vi "Brick setting.vi"(5 "stage":i32, 7 "Ref_brick":refnum<vi>[](array[refnum])) -> (0 "brick(s)":i32, 1 "total_stg":i32, 2 "HP set":i32[](array[numeric]), 3 "Brick_table":refnum<vi>[](array[refnum]))   [LabVIEW 8.6]
uses:
  <vilib>/Utility/file.llb/Read From Spreadsheet File (string).vi
panel:
  in  "Brick 24":bool
  in  "Brick 23":bool
  in  "Brick 22":bool
  in  "Brick 21":bool
  in  "Brick 20":bool
  in  "Brick 19":bool
  in  "Brick 18":bool
  in  "Brick 17":bool
  in  "Brick 16":bool
  in  "Brick 15":bool
  in  "Brick 14":bool
  in  "Brick 13":bool
  in  "Brick 12":bool
  in  "Brick 11":bool
  in  "Brick 10":bool
  in  "Brick 9":bool
  in  "Brick 8":bool
  in  "Brick 7":bool
  in  "Brick 6":bool
  in  "Brick 5":bool
  in  "Brick 4":bool
  in  "Brick 3":bool
  in  "Brick 2":bool
  in  "Brick 1":bool
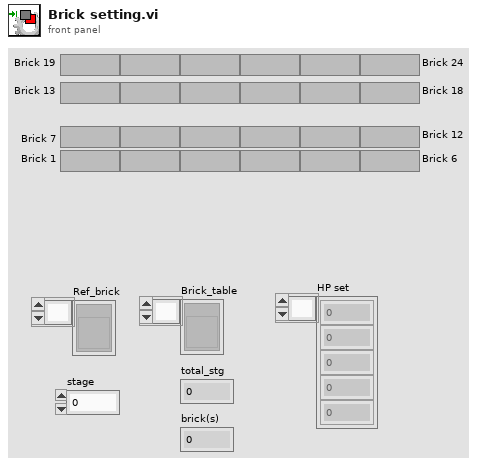
[diagram p1: front panel]
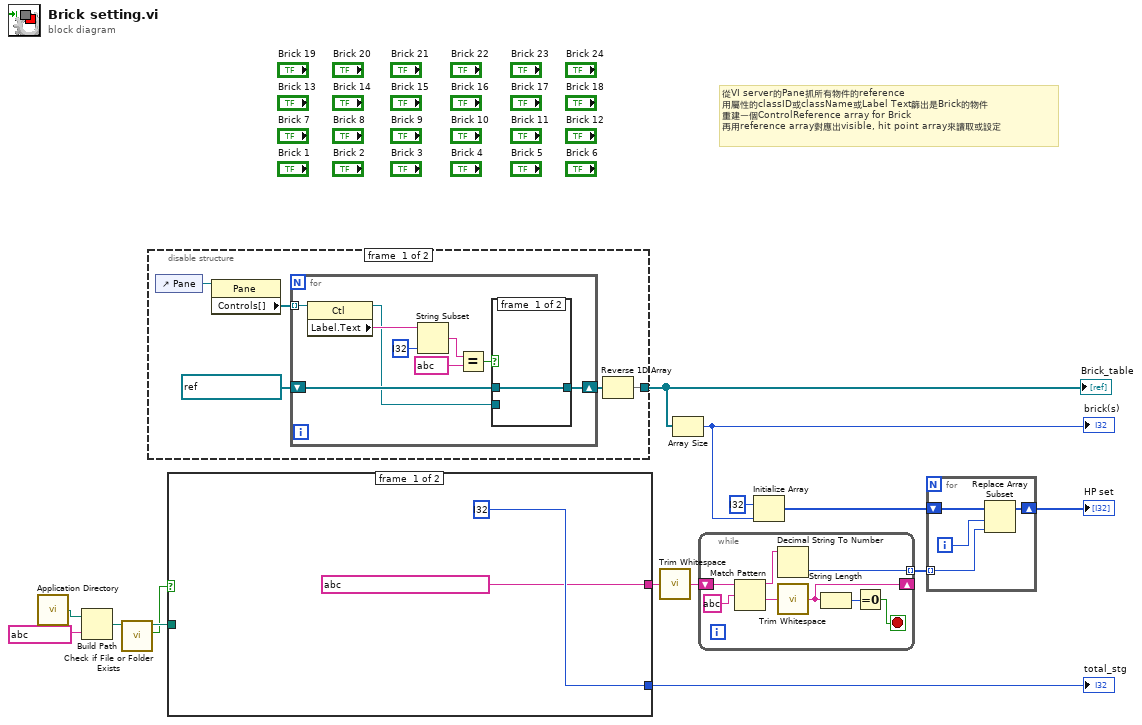
[diagram p0: block diagram]
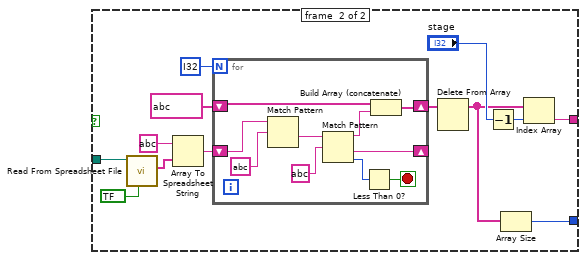
[diagram p2: hidden frame]
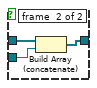
[diagram p3: hidden frame]
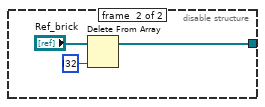
[diagram p4: hidden frame]
diagram:
  # "從VI server的Pane抓所有物件的reference\n用屬性的classID或className或Label Text篩出是Brick的物件\n重建一個ControlReference array for Brick\n再用reference array對應出visible, hit point array來讀取或設定"
  n1 = call <vilib>:"Application Directory.vi"() -> ("Application Directory"=w8:path)
  n2 = Build Path(base path=w8, name or relative path=string ?) -> (appended path=w5:path)
  n3 = call <vilib>:"Check if File or Folder Exists.vi"("path"=w5) -> ("file or folder exists?"=w4:bool, "dup path"=w6:path)  [unwired: 8 in, 1 out]
  n4 = disable-structure shown="Enabled" {
    disable-tunnel: [w15 w33] -> w11
    frame #0 {
      n5 = control-ref of="Pane"() -> (w17:refnum<vi>)
      n6 = property on="Property Node" class="Pane"(reference=w17) -> ("Controls[]"=w19:refnum<vi>[])  [unwired: 1 in, 2 out]
      n7 = for {
        tunnel: w19 -> [w21] mode=indexing
        shift-right: [w23] -> w16
        shift-left: refnum<vi>[] ? -> [w24]
        n8 = property on="Property Node" class="Ctl"(reference=w21) -> (reference out=w20:refnum<vi>, "Label.Text"=w22:string)  [unwired: 1 in, 1 out]
        n9 = String Subset(string=w22, length (rest)=i32 ? ("length (rest)")) -> (substring=w26:string)  [unwired: 1 in]
        n10 = Equal?(x=w26, y=string ?) -> (x = y?=w25:bool)
        n11 = case shown="True" w25 {
          tunnel: w24 -> [w29 w31]
          tunnel: [w29 w32] -> w23
          tunnel: w20 -> [_ w30]
          frame #0 {
          }
          frame #1 {
            n12 = Build Array (concatenate)(w31, w30) -> (w32:refnum<vi>[])
          }
        }
      }
      n13 = Reverse 1D Array(array=w16) -> (reversed array=w15:refnum<vi>[])
    }
    frame #1 {
      n14 = Delete From Array(array="Ref_brick", index=i32 ?) -> (array with subset deleted=w33:refnum<vi>[])  [unwired: 1 in, 1 out]
    }
  }
  "Brick_table" <- w11
  n15 = case shown="True" w4 {
    tunnel: [i32 ? w44] -> w12
    tunnel: w6 -> [_ w43]
    tunnel: [string ? ("spreadsheet string") w42] -> w2
    frame #0 {
    }
    frame #1 {
      n16 = call-poly <vilib>:"Read From Spreadsheet File.vi"("transpose (no:F)"=bool ?, "file path (dialog if empty)"=w43) -> ("first row"=w46:string[])  [unwired: 5 in, 4 out]
      n17 = Array To Spreadsheet String(array=w46, 3:string ? ("format string")) -> (spreadsheet string=w49:string)  [unwired: 1 in]
      n18 = for {
        N: i32 ? -> [_]
        shift-right: [w55] -> w39
        shift-left: string[] ? -> [w53]
        shift-right: [w57] -> _
        shift-left: w49 -> [w56]
        stop <- w52 stop-if-true
        n19 = Match Pattern(string=w56, regular expression=string ?) -> (after substring=w58:string)  [unwired: 1 in, 3 out]
        n20 = Match Pattern(string=w58, regular expression=string ?) -> (before substring=w54:string, after substring=w57:string, offset past match=w51:i32)  [unwired: 1 in, 1 out]
        n21 = Less Than 0?(x=w51) -> (x < 0?=w52:bool)
        n22 = Build Array (concatenate)(w53, w54) -> (w55:string[])
      }
      n23 = Delete From Array(array=w39) -> (array with subset deleted=w38:string[])  [unwired: 2 in, 1 out]
      n24 = Decrement(x="stage") -> (x-1=w40:i32)
      n25 = Array Size(array=w38) -> (size(s)=w44:i32)
      n26 = Index Array(array=w38, index=w40) -> (element=w42:string)
    }
  }
  "total_stg" <- w12
  n27 = call <vilib>:"Trim Whitespace.vi"("string"=w2) -> ("trimmed string"=w1:string)  [unwired: 1 in]
  n28 = Array Size(array=w11) -> (size(s)=w14:i32)
  "brick(s)" <- w14
  n29 = while {
    shift-right: [w64] -> _
    shift-left: w1 -> [w61]
    tunnel: [w62] -> w9 mode=indexing
    stop <- w63 stop-if-true
    n30 = Match Pattern(string=w61, regular expression=string ?) -> (before substring=w67:string, after substring=w65:string)  [unwired: 1 in, 2 out]
    n31 = Decimal String To Number(string=w67) -> (number=w62:i32)  [unwired: 2 in, 1 out]
    n32 = call <vilib>:"Trim Whitespace.vi"("string"=w65) -> ("trimmed string"=w64:string)  [unwired: 1 in]
    n33 = String Length(string=w64) -> (length=w66:i32)
    n34 = Equal To 0?(x=w66) -> (x = 0?=w63:bool)
  }
  n35 = Initialize Array(i32 ? ("element"), w14) -> (w3:i32[])
  n36 = for {
    tunnel: w9 -> [w70] mode=indexing
    shift-right: [w71] -> w13
    shift-left: w3 -> [w72]
    i -> [w69]
    n37 = Replace Array Subset(array=w72, new element=w70, index=w69) -> (w71:i32[])
  }
  "HP set" <- w13
